vi "Read outputs.vi"(8 "error in (no error)":errorcluster, 11 "Power Supply Instrument in":refnum<class "Power Supply Instrument.lvclass">) -> (0 "error out":errorcluster, 2 "outputs":bool[](array[boolean]), 3 "Power Supply Instrument out":refnum<class "Power Supply Instrument.lvclass">)   [LabVIEW 2025, in "Power Supply.lvlib" / "Power Supply Instrument.lvclass"]
uses:
  Power Supply Instrument.lvclass
  Power Supply Instrument.lvclass/Power Supply Instrument.ctl
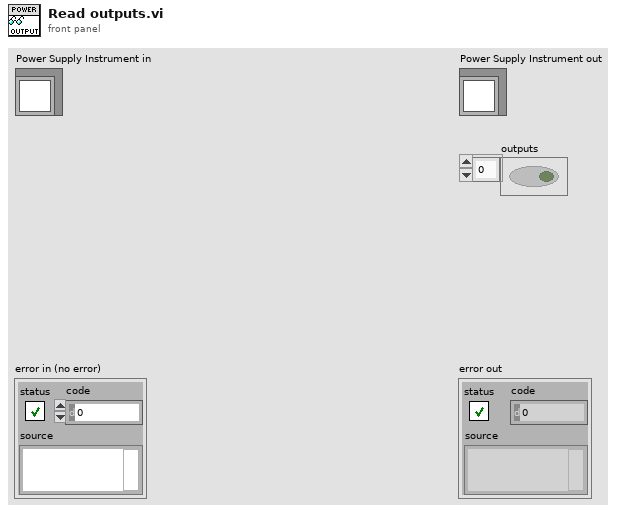
[diagram p1: front panel]
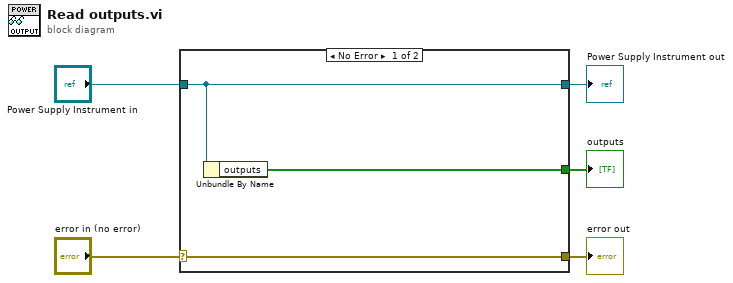
[diagram p0: block diagram]
diagram:
  n1 = case shown="No Error" "error in (no error)" {
    selector: "error in (no error)" -> [w8 w9]
    tunnel: [w8 w9] -> w4
    tunnel: [w7 w10] -> w2
    tunnel: "Power Supply Instrument in" -> [w7 w10]
    tunnel: [w6 _] -> w1
    frame No Error {
      n2 = Unbundle By Name(w7) -> ("outputs"=w6:bool[])
    }
    frame Error {
    }
  }
  "error out" <- w4
  "Power Supply Instrument out" <- w2
  "outputs" <- w1
